vi "mongo_simple_int_command.vi"(8 "arg":i32, 9 "cmdstr":string, 10 "db":string, 11 "conn":T2) -> (0 "result":errorcluster, 3 "out":T1)   [LabVIEW 2013]
uses:
  mongo.ctl
  bson.ctl
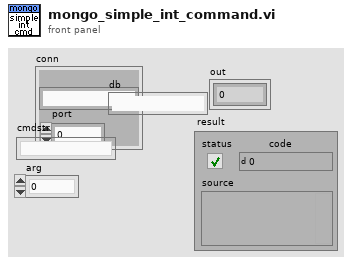
[diagram p1: front panel]
types:
  T1 = typedef "bson.ctl" = cluster{i32}
  T2 = typedef "mongo.ctl" = cluster{"host":string, "port":i32}
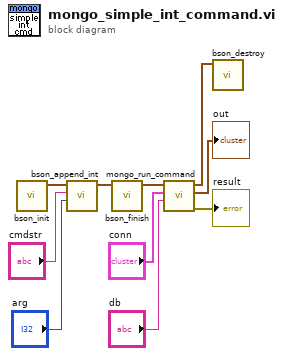
[diagram p0: block diagram]
diagram:
  n1 = call "bson_init.vi"() -> ("cmd out"=w10:T1)  [unwired: 9 in]
  n2 = call "bson_append_int.vi"("arg"="arg", "cmdstr"="cmdstr", "cmd in"=w10) -> ("cmd out"=w9:T1)  [unwired: 8 in]
  n3 = call "bson_finish.vi"("cmd in"=w9) -> ("cmd out"=w8:T1)  [unwired: 10 in]
  n4 = call "mongo_run_command.vi"("db"="db", "conn"="conn", "cmd in"=w8) -> ("result"=→"result":errorcluster, "out"=→"out":T1, "cmd out"=w5:T1)  [unwired: 6 in]
  n5 = call "bson_destroy.vi"("cmd in"=w5) -> ()  [unwired: 10 in, 1 out]
